vi "Get Mouse Click Row.vi"(8 "error in (no error)":errorcluster, 10 "Coords":T1, 11 "Table in":refnum<vi>) -> (0 "error out":errorcluster, 1 "Row":i32, 2 "Column Header Row":bool, 3 "Valid Assert Statement":bool)   [LabVIEW 2016, in "UserInterface.lvlib" / "UserInterface.lvclass"]
uses:
  UserInterface.lvclass
  <vilib>/Utility/miscctls.llb/LVPoint32TypeDef.ctl
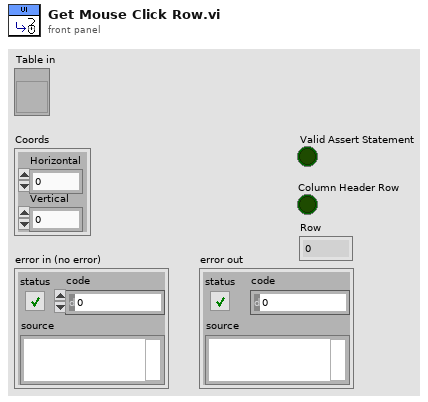
[diagram p1: front panel]
types:
  T1 = typedef "LVPoint32TypeDef.ctl" = cluster{"Horizontal":i32, "Vertical":i32}
  T2 = typedef "LVRowAndColumnTypeDef.ctl" = cluster{"Row":i32, "Column":i32}
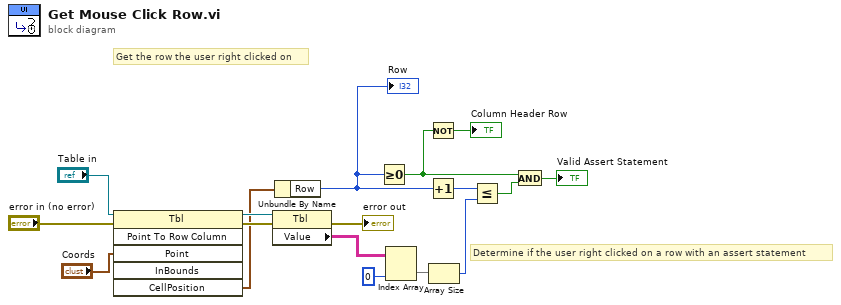
[diagram p0: block diagram]
diagram:
  # "Determine if the user right clicked on a row with an assert statement"
  # "Get the row the user right clicked on"
  n1 = invoke class="Tbl" method="Point To Row Column"(reference="Table in", error in="error in (no error)", "Point"="Coords") -> (reference out=w10:refnum<vi>, error out=w11:errorcluster, "CellPosition"=w4:T2)  [unwired: 3 in, 3 out]
  n2 = property class="Tbl"(reference=w10, error in=w11) -> (error out=→"error out":errorcluster, "Value"=w13:string[][])  [unwired: 1 out]
  n3 = Unbundle By Name(w4) -> ("Row"=w7:i32)
  "Row" <- w7
  n4 = Greater Or Equal To 0?(x=w7) -> (x >= 0?=w2:bool)
  n5 = Index Array(array=w13, index (col)=0 ("disabled index (col)")) -> (element=w15:string[])  [unwired: 1 in]
  n6 = Not(x=w2) -> (.not. x?=→"Column Header Row":bool)
  n7 = Increment(x=w7) -> (x+1=w17:i32)
  n8 = Array Size(array=w15) -> (size(s)=w16:i32)
  n9 = Less Or Equal?(x=w17, y=w16) -> (x <= y?=w9:bool)
  n10 = And(x=w2, y=w9) -> (x .and. y?=→"Valid Assert Statement":bool)
